vi "outputs.vi"() -> ()   [LabVIEW 2019]
doc: "This global variable contains current robot state information and actuator setpoints."
panel:
  out "Force_Low_Gear":bool
  out "Swerve_2_High_Gear_Requested":bool
  out "Swerve_1_High_Gear_Requested":bool
  out "Swerve_3_High_Gear_Requested":bool
  out "Swerve_0_High_Gear_Requested":bool
  out "Swerve_2_Drive_Flip":bool
  out "Swerve_1_Drive_Flip":bool
  out "Swerve_3_Drive_Flip":bool
  out "Swerve_0_Drive_Flip":bool
  out "Swerve_3_Azimuth_Goal (deg)":dbl
  out "Swerve_1_Azimuth_Goal (deg)":dbl
  out "Swerve_2_Azimuth_Goal (deg)":dbl
  out "Swerve_0_Azimuth_Goal (deg)":dbl
  out "Diverting_Power_LEDS":bool
  out "Swerve_Rotation_Command":dbl
  out "Disallowed_Master_States":bool[](array[boolean])
  out "Drive_Mode":T1(ring)
  out "LED_0_Mode":dbl
  out "Intake_Deployed":bool
  out "LimeLight_LED_Mode":i64
  out "LimeLight_Pipeline":i64
  out "Diverting_Power_Compressor":bool
  out "Intake_On":bool
  out "Intake_Power":dbl
  out "Field_Oriented":bool
  out "Confirmed_Master_States":bool[](array[boolean])
  out "Boost_Drive_Current_Limit":bool
  out "Swerve_3_Azimuth_Error (deg)":dbl
  out "Swerve_1_Azimuth_Error (deg)":dbl
  out "Swerve_2_Azimuth_Error (deg)":dbl
  out "Swerve_0_Azimuth_Error (deg)":dbl
  out "Swerve_3_Drive_Command":dbl
  out "Swerve_1_Drive_Command":dbl
  out "Swerve_2_Drive_Command":dbl
  out "Swerve_0_Drive_Command":dbl
  # "--master state controller--"
  # "--drive subsystem--"
  # "--intake and magazine subsystem--"
  # "--power management--"
  # "--LL control--"
  # "--decorations--"
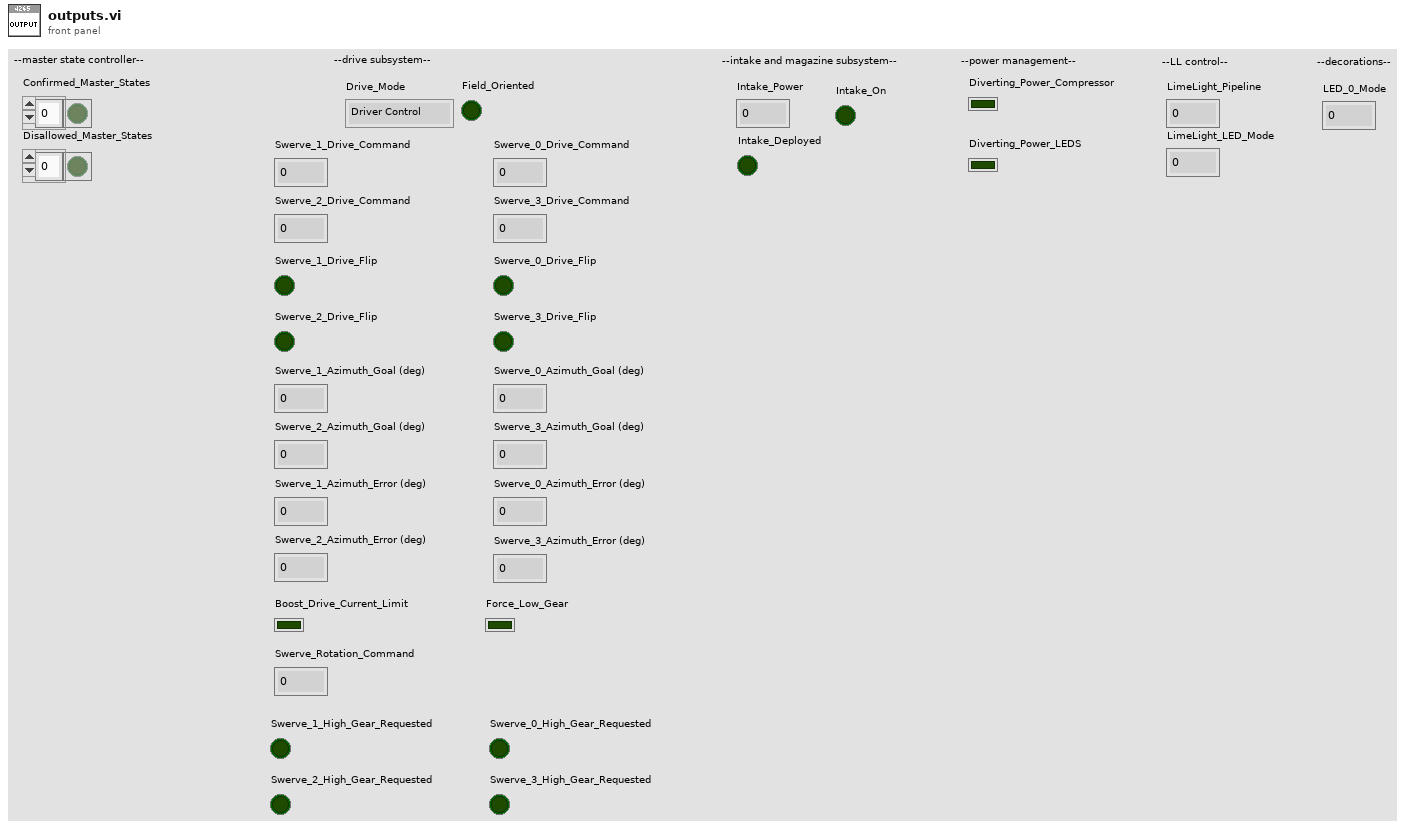
[diagram p1: front panel]
types:
  T1 = enum16{"Driver Control", "Auto Targeting", "Feeder Station"}
diagram:
